vi "GoToBallKeeperSkillVSS.vi"(8 "error in (no error)":errorcluster, 9 "Robot in":refnum<class "Robot.lvclass">, 10 "Game in":refnum<class "Game.lvclass">, 11 "GoToBallKeeperSkillVSS in":refnum<class "GoToBallKeeperSkillVSS.lvclass">) -> (0 "error out":errorcluster, 1 "Robot out":refnum<class "Robot.lvclass">, 3 "GoToBallKeeperSkillVSS out":refnum<class "GoToBallKeeperSkillVSS.lvclass">)   [LabVIEW 2020, in "GoToBallKeeperSkillVSS.lvclass"]
uses:
  GoToBallKeeperSkillVSS.lvclass
  Robot_class/Robot.lvclass
  C:/ROBOIME/SSL_AI/Object_class/Object.lvclass
  Game_class/Game.lvclass
  Object_class/Object.lvclass/Object.ctl
  Game_class/Game.lvclass/Game.ctl
  Team_class/Team.lvclass/Team.ctl
  Robot_class/Robot.lvclass/Robot.ctl
  Game_class/Read BallRef.vi
  Game_class/Read EnemyRef.vi
  Game_class/Read FieldRef.vi
  Team_class/Read RobotRef.vi
  Object_class/Read x.vi
  Object_class/Read y.vi
  Robot_class/Read orientation.vi
  Robot_class/Write dest_orientation.vi
  Object_class/Write x.vi
  Object_class/Write y.vi
  Enemy_class/Enemy.lvclass
  C:/ROBOIME/SSL_AI/Team_class/Team.lvclass
  Ball_class/Ball.lvclass
  Field_class/Field.lvclass
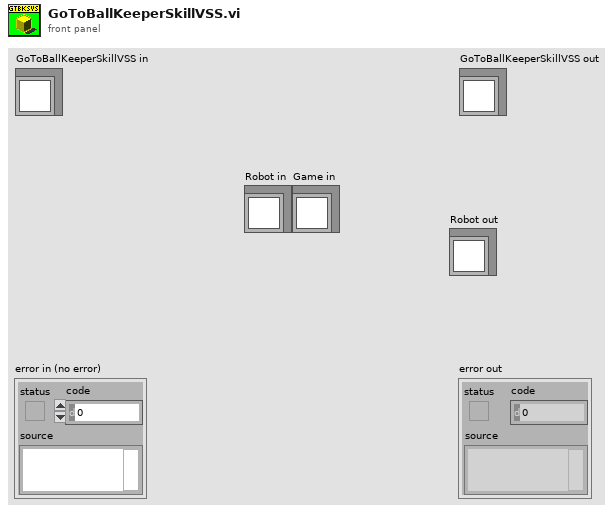
[diagram p1: front panel]
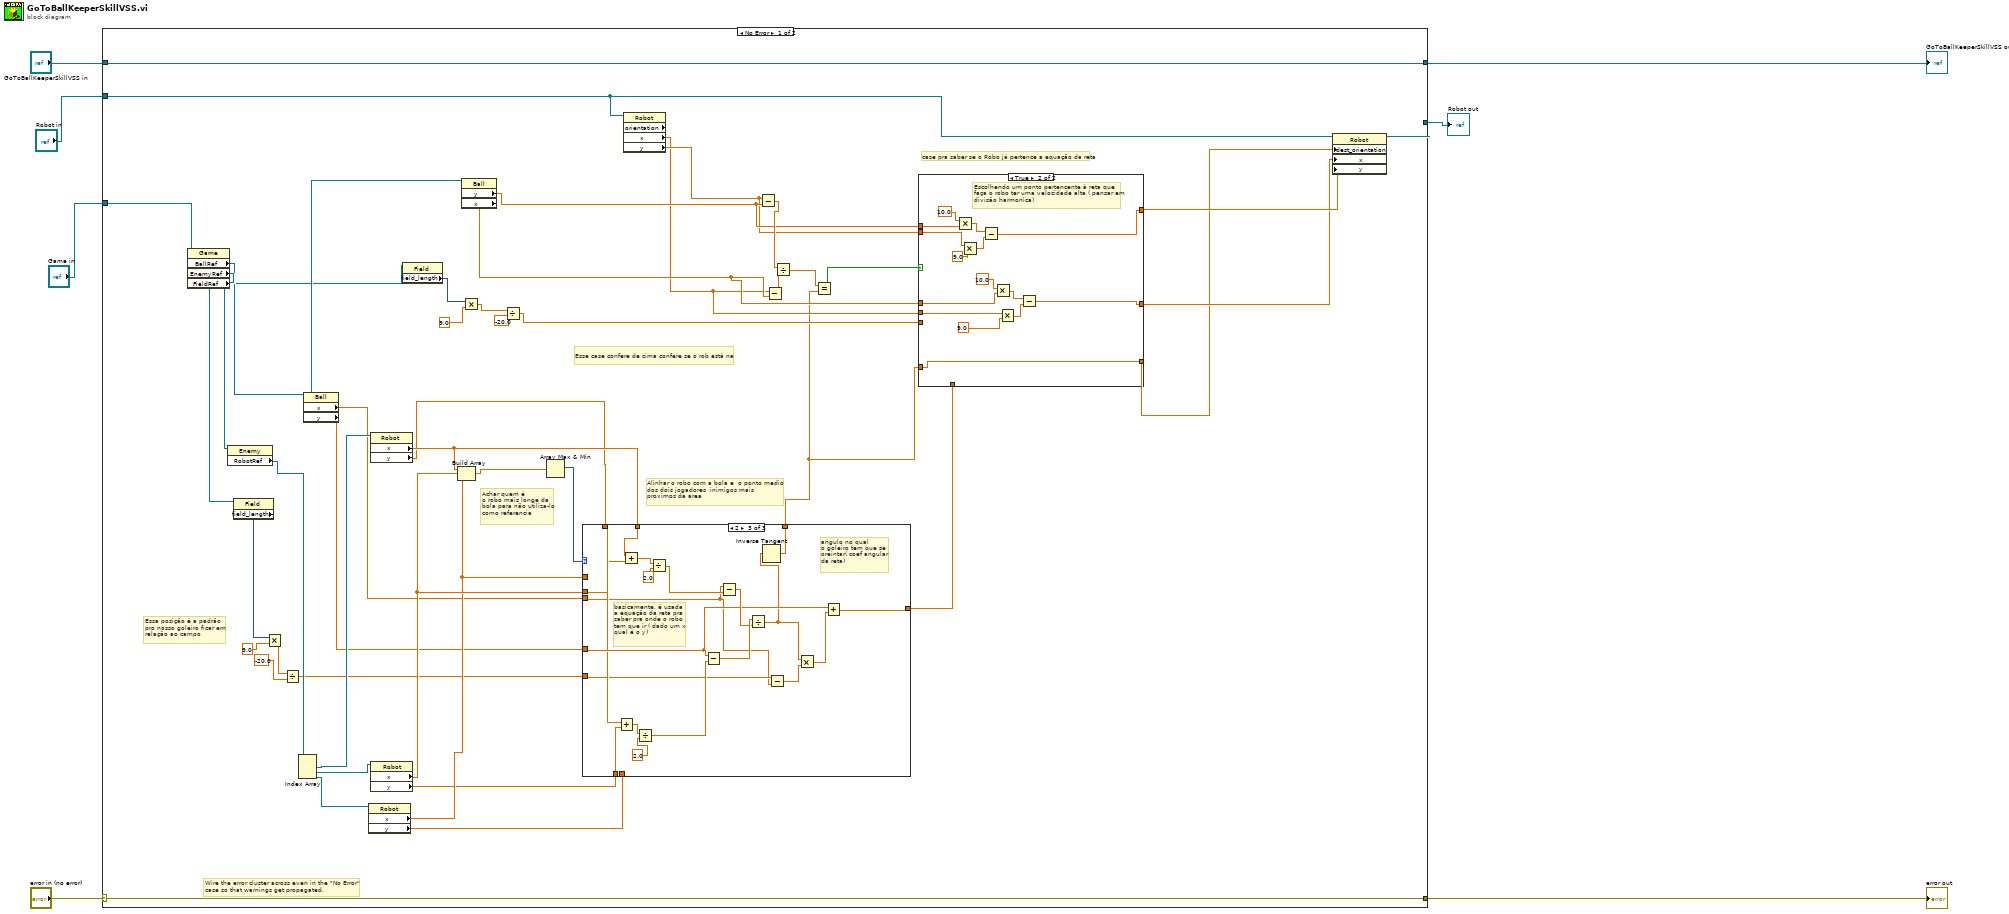
[diagram p0: block diagram]
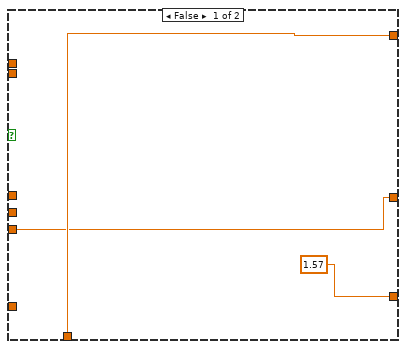
[diagram p2: hidden frame]
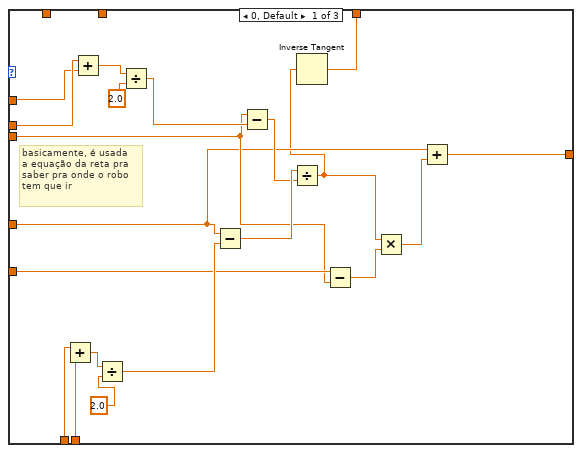
[diagram p3: hidden frame]
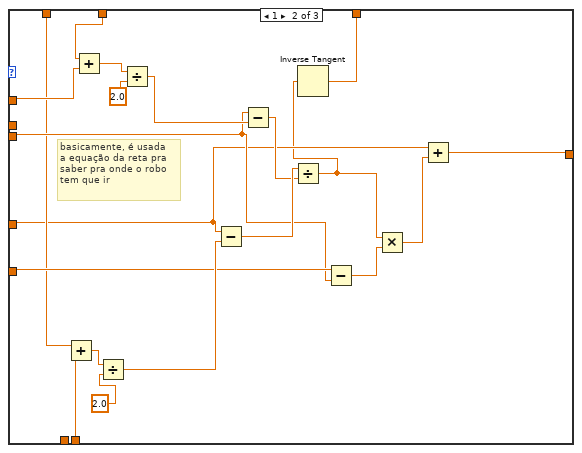
[diagram p4: hidden frame]
diagram:
  n1 = case shown="No Error" "error in (no error)" {
    selector: "error in (no error)" -> [w51 w133]
    tunnel: [w51 w133] -> w6
    tunnel: [w52 w132] -> w4
    tunnel: "GoToBallKeeperSkillVSS in" -> [w52 w132]
    tunnel: "Robot in" -> [w30 w131]
    tunnel: [w50 w131] -> w2
    tunnel: "Game in" -> [w49 _]
    frame No Error {
      # "Esse case confere de cima confere se o rob está na"
      # "Achar quem é \no robo mais longe da\nbola para não utiliza-lo\ncomo referencia"
      # "case pra saber se o Robo já pertence a equação da reta"
      # "Essa posição é a padrão \npro nosso goleiro ficar em\nrelação ao campo"
      # "Alinhar o robo com a bola e  o ponto medio\ndos dois jogadores  inimigos mais\nproximos da area"
      # "Wire the error cluster across even in the \"No Error\"\ncase so that warnings get propagated."
      n2 = property class="Game"(reference=w49) -> ("BallRef"=w21:refnum<class "Ball.lvclass">, "EnemyRef"=w44:refnum<class "Enemy.lvclass">, "FieldRef"=w16:refnum<class "Field.lvclass">)  [unwired: 1 in, 2 out]
      n3 = property class="Enemy"(reference=w44) -> ("RobotRef"=w48:refnum<class "Robot.lvclass">[])  [unwired: 1 in, 2 out]
      n4 = property class="Field"(reference=w16) -> ("field_length"=w37:i32)  [unwired: 1 in, 2 out]
      n5 = Multiply(x=w37, y=9.0) -> (x*y=w35:dbl)
      n6 = Divide(x=w35, y=-20.0) -> (x/y=w33:dbl)
      n7 = Index Array(array=w48) -> (element #1=w47:refnum<class "Robot.lvclass">, element #2=w46:refnum<class "Robot.lvclass">, element #3=w45:refnum<class "Robot.lvclass">)  [unwired: 3 in]
      n8 = property class="Ball"(reference=w21) -> ("x"=w31:dbl, "y"=w38:dbl)  [unwired: 1 in, 2 out]
      n9 = property class="Robot"(reference=w45) -> ("x"=w39:dbl, "y"=w41:dbl)  [unwired: 1 in, 2 out]
      n10 = property class="Robot"(reference=w47) -> ("x"=w29:dbl, "y"=w28:dbl)  [unwired: 1 in, 2 out]
      n11 = property class="Robot"(reference=w46) -> ("x"=w40:dbl, "y"=w32:dbl)  [unwired: 1 in, 2 out]
      n12 = property class="Field"(reference=w16) -> ("field_length"=w14:i32)  [unwired: 1 in, 2 out]
      n13 = Build Array(w29, w40, w39) -> (w43:dbl[])
      n14 = property class="Ball"(reference=w21) -> ("y"=w19:dbl, "x"=w20:dbl)  [unwired: 1 in, 2 out]
      n15 = Multiply(x=w14, y=9.0) -> (x*y=w13:dbl)
      n16 = Divide(x=w13, y=-20.0) -> (x/y=w10:dbl)
      n17 = Array Max & Min(array=w43) -> (max index (indices)=w42:i32)  [unwired: 3 out]
      n18 = case shown="2" w42 {
        tunnel: w41 -> [w90 w102 _]
        tunnel: w40 -> [w87 _ w113]
        tunnel: w39 -> [w86 w100 _]
        tunnel: w38 -> [w73 w94 w120]
        tunnel: w31 -> [w74 w97 w116]
        tunnel: w33 -> [w81 w101 w117]
        tunnel: [w78 w93 w115] -> w23
        tunnel: w32 -> [w77 _ w114]
        tunnel: w29 -> [_ w96 w119]
        tunnel: w28 -> [_ w95 w118]
        tunnel: [w71 w91 w111] -> w9
        frame 0, Default {
          # "basicamente, é usada\na equação da reta pra \nsaber pra onde o robo \ntem que ir"
          n19 = Add(x=w77, y=w90) -> (x+y=w89:dbl)
          n20 = Add(x=w87, y=w86) -> (x+y=w84:dbl)
          n21 = Divide(x=w89, y=2.0) -> (x/y=w83:dbl)
          n22 = Divide(x=w84, y=2.0) -> (x/y=w82:dbl)
          n23 = Subtract(x=w73, y=w83) -> (x-y=w76:dbl)
          n24 = Subtract(x=w74, y=w82) -> (x-y=w75:dbl)
          n25 = Divide(x=w76, y=w75) -> (x/y=w72:dbl)
          n26 = Inverse Tangent(1:w72) -> (0:w71:dbl)
          n27 = Subtract(x=w81, y=w74) -> (x-y=w80:dbl)
          n28 = Multiply(x=w72, y=w80) -> (x*y=w79:dbl)
          n29 = Add(x=w73, y=w79) -> (x+y=w78:dbl)
        }
        frame 1 {
          # "basicamente, é usada\na equação da reta pra \nsaber pra onde o robo \ntem que ir"
          n30 = Add(x=w95, y=w102) -> (x+y=w110:dbl)
          n31 = Add(x=w96, y=w100) -> (x+y=w107:dbl)
          n32 = Divide(x=w110, y=2.0) -> (x/y=w106:dbl)
          n33 = Divide(x=w107, y=2.0) -> (x/y=w105:dbl)
          n34 = Subtract(x=w94, y=w106) -> (x-y=w99:dbl)
          n35 = Subtract(x=w97, y=w105) -> (x-y=w98:dbl)
          n36 = Divide(x=w99, y=w98) -> (x/y=w92:dbl)
          n37 = Inverse Tangent(1:w92) -> (0:w91:dbl)
          n38 = Subtract(x=w101, y=w97) -> (x-y=w104:dbl)
          n39 = Multiply(x=w92, y=w104) -> (x*y=w103:dbl)
          n40 = Add(x=w94, y=w103) -> (x+y=w93:dbl)
        }
        frame 2 {
          # "angulo no qual \no goleiro tem que se \noreintar( coef angular\nda reta)"
          # "basicamente, é usada\na equação da reta pra \nsaber pra onde o robo \ntem que ir ( dado um x\nqual é o y)"
          n41 = Add(x=w118, y=w114) -> (x+y=w130:dbl)
          n42 = Add(x=w119, y=w113) -> (x+y=w127:dbl)
          n43 = Divide(x=w130, y=2.0) -> (x/y=w126:dbl)
          n44 = Divide(x=w127, y=2.0) -> (x/y=w125:dbl)
          n45 = Subtract(x=w120, y=w126) -> (x-y=w122:dbl)
          n46 = Subtract(x=w116, y=w125) -> (x-y=w121:dbl)
          n47 = Divide(x=w122, y=w121) -> (x/y=w112:dbl)
          n48 = Inverse Tangent(1:w112) -> (0:w111:dbl)
          n49 = Subtract(x=w117, y=w116) -> (x-y=w124:dbl)
          n50 = Multiply(x=w112, y=w124) -> (x*y=w123:dbl)
          n51 = Add(x=w120, y=w123) -> (x+y=w115:dbl)
        }
      }
      n52 = property class="Robot" props=["orientation", "x", "y"](reference=w30) -> ("x"=w11:dbl, "y"=w18:dbl)  [unwired: 1 in, 3 out]
      n53 = Subtract(x=w18, y=w19) -> (x-y=w27:dbl)
      n54 = Subtract(x=w11, y=w20) -> (x-y=w26:dbl)
      n55 = Divide(x=w27, y=w26) -> (x/y=w25:dbl)
      n56 = Equal?(x=w25, y=w9) -> (x = y?=w24:bool)
      n57 = case shown="True" w24 {
        tunnel: w23 -> [w55 _]
        tunnel: [w55 w58] -> w22
        tunnel: w20 -> [_ w69]
        tunnel: w11 -> [_ w67]
        tunnel: w19 -> [_ w62]
        tunnel: w18 -> [_ w61]
        tunnel: [w54 w57] -> w17
        tunnel: w10 -> [w54 _]
        tunnel: w9 -> [_ w56]
        tunnel: [1.57 w56] -> w8
        frame False {
        }
        frame True {
          # "Escolhendo um ponto pertencente à reta que\nfaça o robo ter uma velocidade alta ( pensar em\ndivisão harmonica)"
          n58 = Multiply(x=10.0, y=w62) -> (x*y=w64:dbl)
          n59 = Multiply(x=w61, y=9.0) -> (x*y=w59:dbl)
          n60 = Subtract(x=w64, y=w59) -> (x-y=w58:dbl)
          n61 = Multiply(x=10.0, y=w69) -> (x*y=w68:dbl)
          n62 = Multiply(x=w67, y=9.0) -> (x*y=w63:dbl)
          n63 = Subtract(x=w68, y=w63) -> (x-y=w57:dbl)
        }
      }
      n64 = property class="Robot"(reference=w30, "dest_orientation"=w8, "x"=w17, "y"=w22) -> (reference out=w50:refnum<class "Robot.lvclass">)  [unwired: 1 in, 1 out]
    }
    frame Error {
    }
  }
  "error out" <- w6
  "GoToBallKeeperSkillVSS out" <- w4
  "Robot out" <- w2
